vi "ToggleAngle.vi"(8 "error in (no error)":errorcluster) -> (0 "error out":errorcluster)   [LabVIEW 2013]
panel:
  in  "Low Exit Angle":dbl
  in  "High Exit Angle":dbl
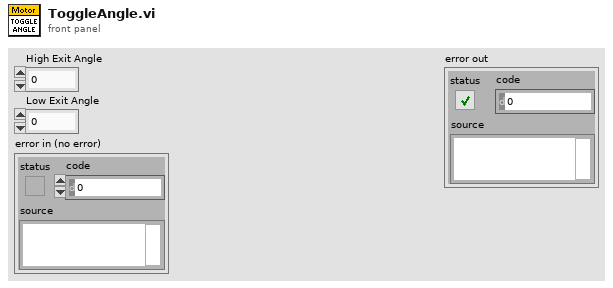
[diagram p1: front panel]
types:
  T1 = typedef "WPI_MotorControlDeviceRef.ctl" = cluster{"DeviceStatus":errorcluster, "Type":enum16{"PWM", "CAN"}, "PWM":cluster{"Digital Module":T2, "PWM Channel":T3, "DeadBand":T4}, "CAN":cluster{"Device Number":u8, "Control Mode":T5, "Semaphore":T6, "Max Vout":dbl}, "Invert":bool, "TransformRef":T7, "InvTransformRef":T7}
  T2 = typedef "FPGA_TypedefDigitalModule.ctl" = enum16{"Digital Module 1", "Digital Module 2"}
  T3 = typedef "FPGA_DIOPWMChannel.ctl" = enum8{"PWM 1", "PWM 2", "PWM 3", "PWM 4", "PWM 5", "PWM 6", "PWM 7", "PWM 8", "PWM 9", "PWM 10", "Invalid"}
  T4 = typedef "WPI_PWMDeadband.ctl" = cluster{"Name":string, "maxPositivePwm":i32, "minPositivePwm":i32, "centerPwm":i32, "maxNegativePwm":i32, "minNegativePwm":i32, "angularRange":u16}
  T5 = typedef "WPI_CANJaguar_ControlMode.ctl" = enum8{"Percent VBus", "Current", "Speed", "Position", "Voltage"}
  T6 = typedef "Semaphore RefNum" = refnum<k1>
  T7 = typedef "WPI_PWMTransform_ConPane.ctl" = refnum<vi>
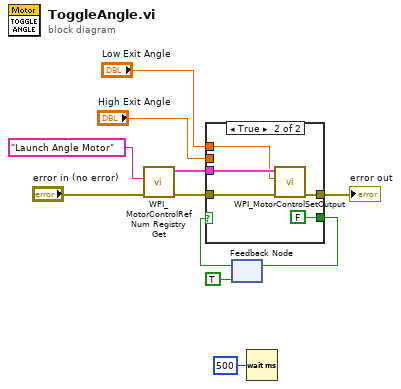
[diagram p0: block diagram]
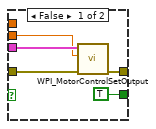
[diagram p2: hidden frame]
diagram:
  n1 = call <vilib>:"WPI_MotorControlRefNum Registry Get.vi"("error in (no error)"="error in (no error)", "refnum name"="Launch Angle Motor") -> ("error out"=w7:errorcluster, "MotorControlDevRef"=w8:T1)  [unwired: 8 in]
  n2 = feedback #1(TRUE) -> (w10:bool)
  n3 = case shown="True" w10 {
    tunnel: [TRUE FALSE] -> w11
    tunnel: w8 -> [w14 w20]
    tunnel: w7 -> [w15 w19]
    tunnel: "High Exit Angle" -> [w13 _]
    tunnel: [w12 w17] -> w3
    tunnel: "Low Exit Angle" -> [_ w18]
    frame False {
      n4 = call <vilib>:"WPI_MotorControlSetOutput.vi"("error in (no error)"=w15, "Output"=w13, "MotorControlDevRef"=w14) -> ("error out"=w12:errorcluster)  [unwired: 6 in, 2 out]
    }
    frame True {
      n5 = call <vilib>:"WPI_MotorControlSetOutput.vi"("error in (no error)"=w19, "Output"=w18, "MotorControlDevRef"=w20) -> ("error out"=w17:errorcluster)  [unwired: 6 in, 2 out]
    }
  }
  "error out" <- w3
  n6 = feedback-in #1(w11) -> ()
  n7 = Wait (ms)(milliseconds to wait=u32 500) -> ()  [unwired: 1 out]
